vi "WriteData.vi"(11 "Array":u16[](array[numeric])) -> (3 "Table":picture)   [LabVIEW 2019]
panel:
  in  "[user-specified font]":T1={"Font Name:"="Arial", "Size"=15, "Strikeout?"=FALSE, "Italic?"=FALSE, "Underline?"=FALSE, "Outline?"=FALSE, "Shadow?"=FALSE, "Bold?"=TRUE}
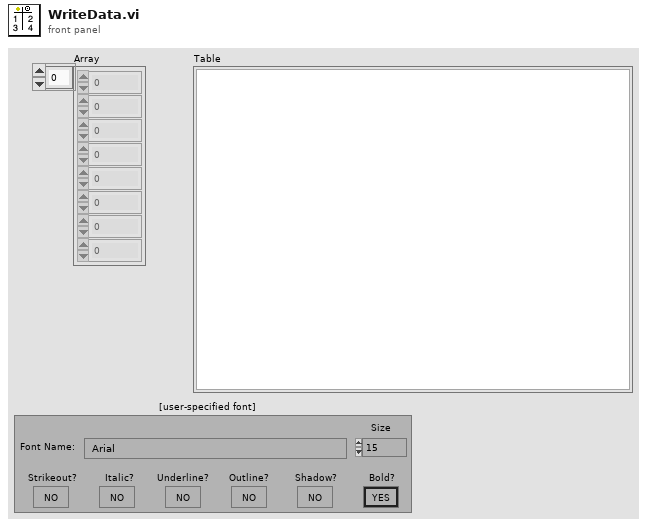
[diagram p1: front panel]
types:
  T1 = cluster{"Font Name:":string, "Size":i16, "Strikeout?":bool, "Italic?":bool, "Underline?":bool, "Outline?":bool, "Shadow?":bool, "Bold?":bool}
  T2 = enum16{"User-specified Font", "Application Font", "System Font", "Dialog Font"}
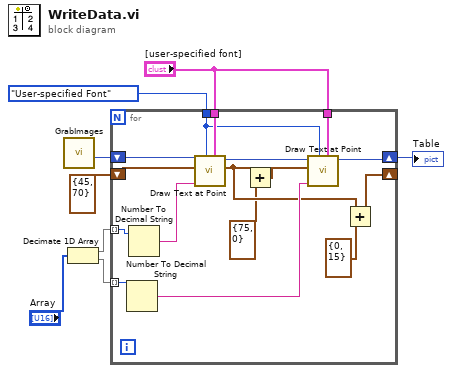
[diagram p0: block diagram]
diagram:
  n1 = call "GrabImages.vi"() -> ("Table"=w7:picture)  [unwired: 8 in, 3 out]
  n2 = Decimate 1D Array("Array") -> (w5:u16[], w4:u16[])
  n3 = for {
    shift-right: [w21] -> w8
    shift-left: w7 -> [w23]
    tunnel: w5 -> [w20] mode=indexing
    tunnel: w4 -> [w19] mode=indexing
    shift-right: [w14] -> _
    shift-left: cluster{"x":i16, "y":i16} {"x"=45, "y"=70} ("origin") -> [w15]
    tunnel: "[user-specified font]" -> [w11]
    tunnel: "[user-specified font]" -> [w10]
    tunnel: T2."User-specified Font" ("desired font(Application)") -> [w9]
    n4 = Number To Decimal String(number=w19) -> (decimal integer string=w18:string)  [unwired: 1 in]
    n5 = Number To Decimal String(number=w20) -> (decimal integer string=w17:string)  [unwired: 1 in]
    n6 = call <vilib>:"Draw Text at Point.vi"("[user-specified font]"=w11, "desired font(Application)"=w9, "text"=w17, "origin"=w15, "picture"=w23) -> ("new picture"=w22:picture)  [unwired: 5 in, 1 out]
    n7 = Add(x=w15, y=cluster{"x":i16, "y":i16} {"x"=75, "y"=0} ("origin")) -> (x+y=w16:cluster{"x":i16, "y":i16})
    n8 = call <vilib>:"Draw Text at Point.vi"("[user-specified font]"=w10, "desired font(Application)"=w9, "text"=w18, "origin"=w16, "picture"=w22) -> ("new picture"=w21:picture)  [unwired: 5 in, 1 out]
    n9 = Add(x=w15, y=cluster{"x":i16, "y":i16} {"x"=0, "y"=15} ("origin")) -> (x+y=w14:cluster{"x":i16, "y":i16})
  }
  "Table" <- w8
